vi "Get Control Refnums No Error.vi"(8 "error in (no error)":errorcluster, 9 "Names":string[](array[string]), 10 "viref Block":refnum<vi>, 11 "Controls[]":refnum<vi>[](array[refnum])) -> (0 "error out":errorcluster, 2 "Indices":u32[](array[numeric]), 3 "Refs Output":refnum<vi>[](array[refnum]))   [LabVIEW 2017]
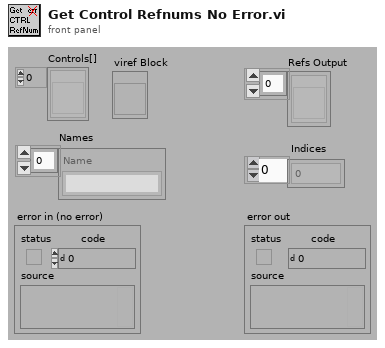
[diagram p1: front panel]
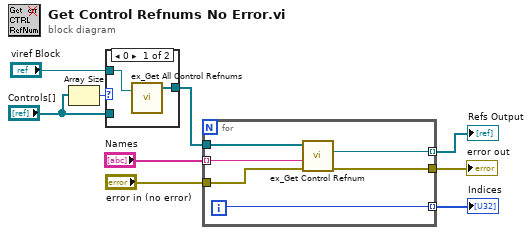
[diagram p0: block diagram]
diagram:
  n1 = Array Size(array="Controls[]") -> (size(s)=w6:i32)
  n2 = case shown="0" w6 {
    tunnel: "Controls[]" -> [_ w12]
    tunnel: "viref Block" -> [w11 _]
    tunnel: [w10 w12] -> w4
    frame 0 {
      n3 = call <vilib>:"ex_Get All Control Refnums.vi"("viref Express VI"=w11) -> ("All Controls[]"=w10:refnum<vi>[])  [unwired: 2 in, 1 out]
    }
    frame 1, Default {
    }
  }
  n4 = for {
    tunnel: "Names" -> [w18] mode=indexing
    tunnel: [w15] -> w8 mode=indexing
    tunnel: w4 -> [w14]
    tunnel: [w13] -> w3 mode=indexing
    tunnel: "error in (no error)" -> [w17]
    tunnel: [w16] -> w1
    i -> [w13]
    n5 = call <vilib>:"ex_Get Control Refnum.vi"("error in (no error)"=w17, "Name"=w18, "Controls[]"=w14) -> ("error out"=w16:errorcluster, "Ctl Refnum"=w15:refnum<vi>)  [unwired: 7 in]
  }
  "Refs Output" <- w8
  "error out" <- w1
  "Indices" <- w3
